vi "Motor Control.vi"(8 "Error In":errorcluster, 9 "Case Event":T1, 10 "Cluster":T2, 11 "VISA resource name":refnum<visa-resource-name>) -> (0 "Error Out":errorcluster, 3 "Serial Response":string)   [LabVIEW 2017]
uses:
  EventCase.ctl
panel:
  in  "SEND":bool
  in  "Stop Button":bool
  out "Parameter String":string
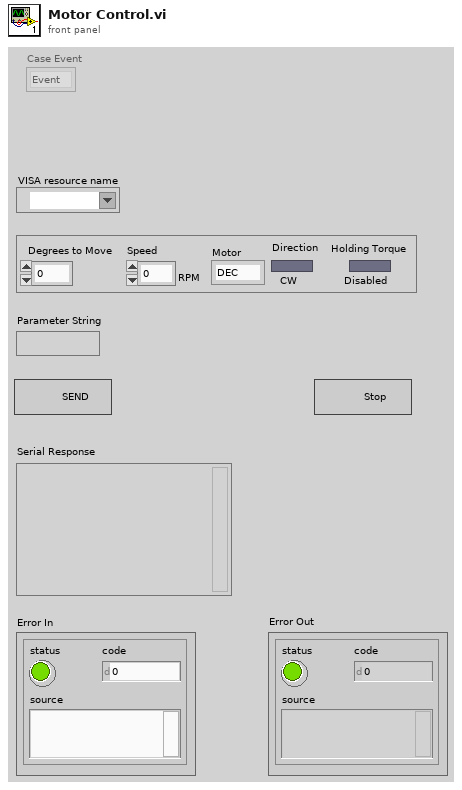
[diagram p1: front panel]
types:
  T1 = typedef "EventCase.ctl" = enum16{"Event", "Serial Write", "Wait", "Serial Read", "Stop"}
  T2 = cluster{"Degrees to Move":dbl, "Speed":i32, "Motor":enum16{"DEC", "RA"}, "Direction":bool, "Holding Torque":bool}
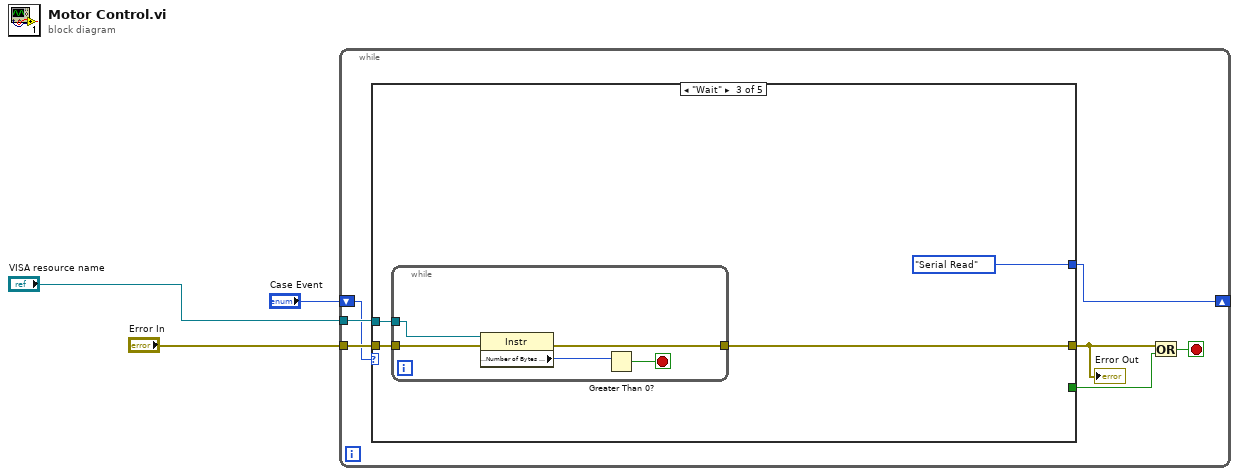
[diagram p0: block diagram]
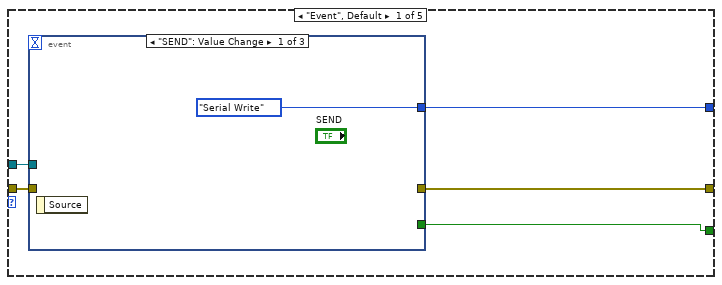
[diagram p2: hidden frame]
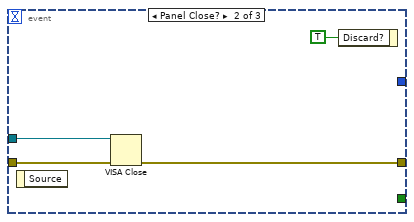
[diagram p3: hidden frame]
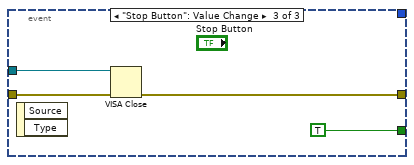
[diagram p4: hidden frame]
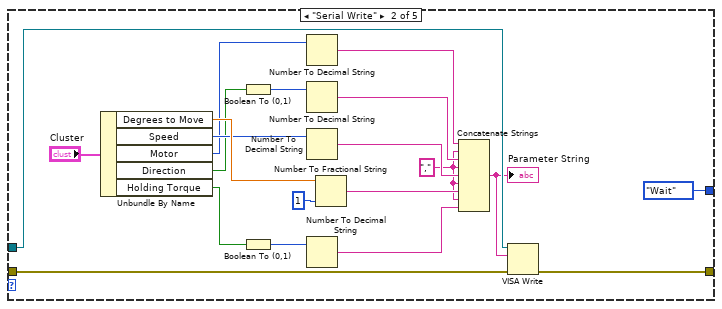
[diagram p5: hidden frame]
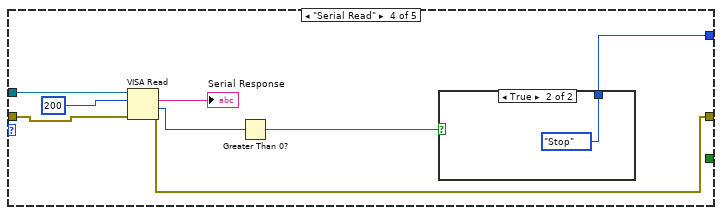
[diagram p6: hidden frame]
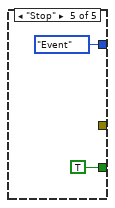
[diagram p8: hidden frame]
diagram:
  n1 = while {
    tunnel: "VISA resource name" -> [w7]
    tunnel: "Error In" -> [w6]
    shift-right: [w4] -> _
    shift-left: "Case Event" -> [w5]
    stop <- w10 stop-if-true
    n2 = case shown="\"Wait\"" w5 {
      tunnel: [w15 w28 w46 w54 _] -> w9
      tunnel: [w14 _ _ _ TRUE] -> w8
      tunnel: w7 -> [w12 w30 w48 w61 _]
      tunnel: w6 -> [w13 w29 w47 w55 _]
      tunnel: [w11 EventCase."Wait" ("Case Event") EventCase."Serial Read" ("Case Event") w56 EventCase."Event" ("Case Event")] -> w4
      frame "Event", Default {
        n3 = event shown="[0] \"SEND\": Value Change" {
          selector: _ -> [_ _ _]
          dyn-events: _ -> [_ _ _]
          timeout: _ -> [_ _ _]
          tunnel: [_ w19 w23] -> w15
          tunnel: [_ _ TRUE] -> w14
          tunnel: w13 -> [_ w18 w22]
          tunnel: w12 -> [_ w17 w21]
          tunnel: [EventCase."Serial Write" ("Case Event") _ _] -> w11
          event "SEND": Value Change {
            n4 = event-data() -> ()  [unwired: 1 in, 1 out]
          }
          event Panel Close? {
            n5 = event-data() -> ()  [unwired: 1 in, 1 out]
            n6 = VISA Close(VISA resource name=w17, error in (no error)=w18) -> (error out=w19:errorcluster)
            n7 = event-data("Discard?"=TRUE) -> ()  [unwired: 1 in, 1 out]
          }
          event "Stop Button": Value Change {
            n8 = event-data() -> ()  [unwired: 1 in, 2 out]
            n9 = VISA Close(VISA resource name=w21, error in (no error)=w22) -> (error out=w23:errorcluster)
          }
        }
      }
      frame "Serial Write" {
        w31 = ","
        n10 = Unbundle By Name("Cluster") -> ("Degrees to Move"=w43:dbl, "Speed"=w42:i32, "Motor"=w40:enum16{"DEC", "RA"}, "Direction"=w41:bool, "Holding Torque"=w44:bool)
        n11 = Boolean To (0,1)(Boolean=w41) -> (0, 1=w39:i16)
        n12 = Boolean To (0,1)(Boolean=w44) -> (0, 1=w38:i16)
        n13 = Number To Decimal String(number=w40) -> (decimal integer string=w37:string)  [unwired: 1 in]
        n14 = Number To Decimal String(number=w39) -> (decimal integer string=w36:string)  [unwired: 1 in]
        n15 = Number To Decimal String(number=w42) -> (decimal integer string=w35:string)  [unwired: 1 in]
        n16 = Number To Decimal String(number=w38) -> (decimal integer string=w33:string)  [unwired: 1 in]
        n17 = Number To Fractional String(number=w43, precision (6)=i16 1) -> (F-format string=w34:string)  [unwired: 2 in]
        n18 = Concatenate Strings(w37, w31, w36, w31, w35, w31, w34, w31, w33) -> (w27:string)
        "Parameter String" <- w27
        n19 = VISA Write(VISA resource name=w30, write buffer=w27, error in (no error)=w29) -> (error out=w28:errorcluster)  [unwired: 2 out]
      }
      frame "Wait" {
        n20 = while {
          tunnel: w48 -> [w53]
          tunnel: w47 -> [w52]
          tunnel: [w51] -> w46
          stop <- w49 stop-if-true
          n21 = property class="Instr"(reference=w53, error in=w52) -> (error out=w51:errorcluster, "Serial Settings:Number of Bytes at Serial Port"=w50:u32)  [unwired: 1 out]
          n22 = Greater Than 0?(x=w50) -> (x > 0?=w49:bool)
        }
      }
      frame "Serial Read" {
        n23 = VISA Read(VISA resource name=w61, byte count=u32 200, error in (no error)=w55) -> (read buffer=→"Serial Response":string, return count=w58:u32, error out=w54:errorcluster)  [unwired: 1 out]
        n24 = Greater Than 0?(x=w58) -> (x > 0?=w57:bool)
        n25 = case shown="True" w57 {
          tunnel: [_ EventCase."Stop" ("Case Event")] -> w56
          frame False {
          }
          frame True {
          }
        }
      }
      frame "Stop" {
      }
    }
    "Error Out" <- w9
    n26 = Or(x=w9, y=w8) -> (x .or. y?=w10:bool)
  }
